vi "Initialize Global Stop.vi"(8 "error in (no error)":errorcluster) -> (0 "error out":errorcluster {"code" min=0 max=0}, 3 "vi reference":T1)   [LabVIEW 2013, in "FPGA Addon Engine.lvlib" / "Stop FG.lvlib"]
uses:
  Stop FG.lvlib
  Stop Global Ref.ctl
  Stop Global Commands.ctl
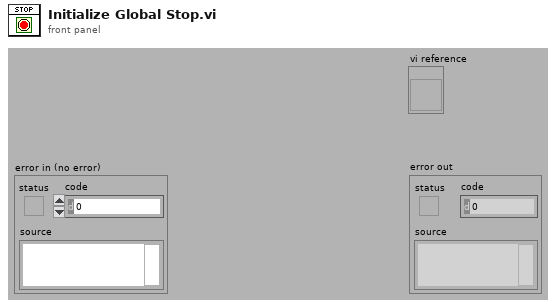
[diagram p1: front panel]
types:
  T1 = typedef "FPGA Addon Engine.lvlib/Stop FG.lvlib/Stop Global Ref.ctl" = refnum<vi>
  T2 = typedef "FPGA Addon Engine.lvlib/Stop FG.lvlib/Stop Global Commands.ctl" = enum16{"Write", "Read", "Reset"}
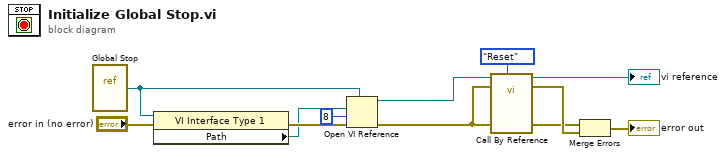
[diagram p0: block diagram]
diagram:
  n1 = vi-ref "Global Stop.vi"() -> (w12:refnum<vi>)
  n2 = property class="VI Interface Type 1"(reference=w12, error in="error in (no error)") -> (error out=w10:errorcluster, "Path"=w7:path)  [unwired: 1 out]
  n3 = Open VI Reference(type specifier VI Refnum (for type only)=w12, vi path=w7, options=8, error in (no error)=w10) -> (vi reference=w6:refnum<vi>, error out=w2:errorcluster)  [unwired: 2 in]
  n4 = call-by-ref "?"(reference=w6, error in=w2, "Command"=Stop_Global_Commands."Reset", 8:"error in (no error)"=w2) -> (reference out=→"vi reference":refnum<vi>, error out=w5:errorcluster, 0:"error out"=w3:errorcluster)  [unwired: 7 in, 2 out]
  n5 = Merge Errors(w3, w5) -> (→"error out":errorcluster)
